vi "GXMLTest.vi"() -> ()   [LabVIEW 2015]
uses:
  <vilib>/NI/GXML/_subVIs/GXML SearchParser/Search Parser.vi
  <vilib>/NI/GXML/GXML.lvlib
panel:
  in  "Write?":bool
  in  "XML File Path":path=path "C:/SoftwareDevelopment/Workspace_2017/XpathTest/src/xpathTest/gxmlExport.xml"
  out "Concatenated GXML String":string
  in  "PID":T1
  in  "encoder":T2
  in  "limit":T3
  in  "template":T4
  in  "motor":T5
  in  "xmlEntries":enum32{"IntakeLift", "ChooChoo"}(tab)
  in  "IntakeLift":T4
  in  "ChooChoo":T4
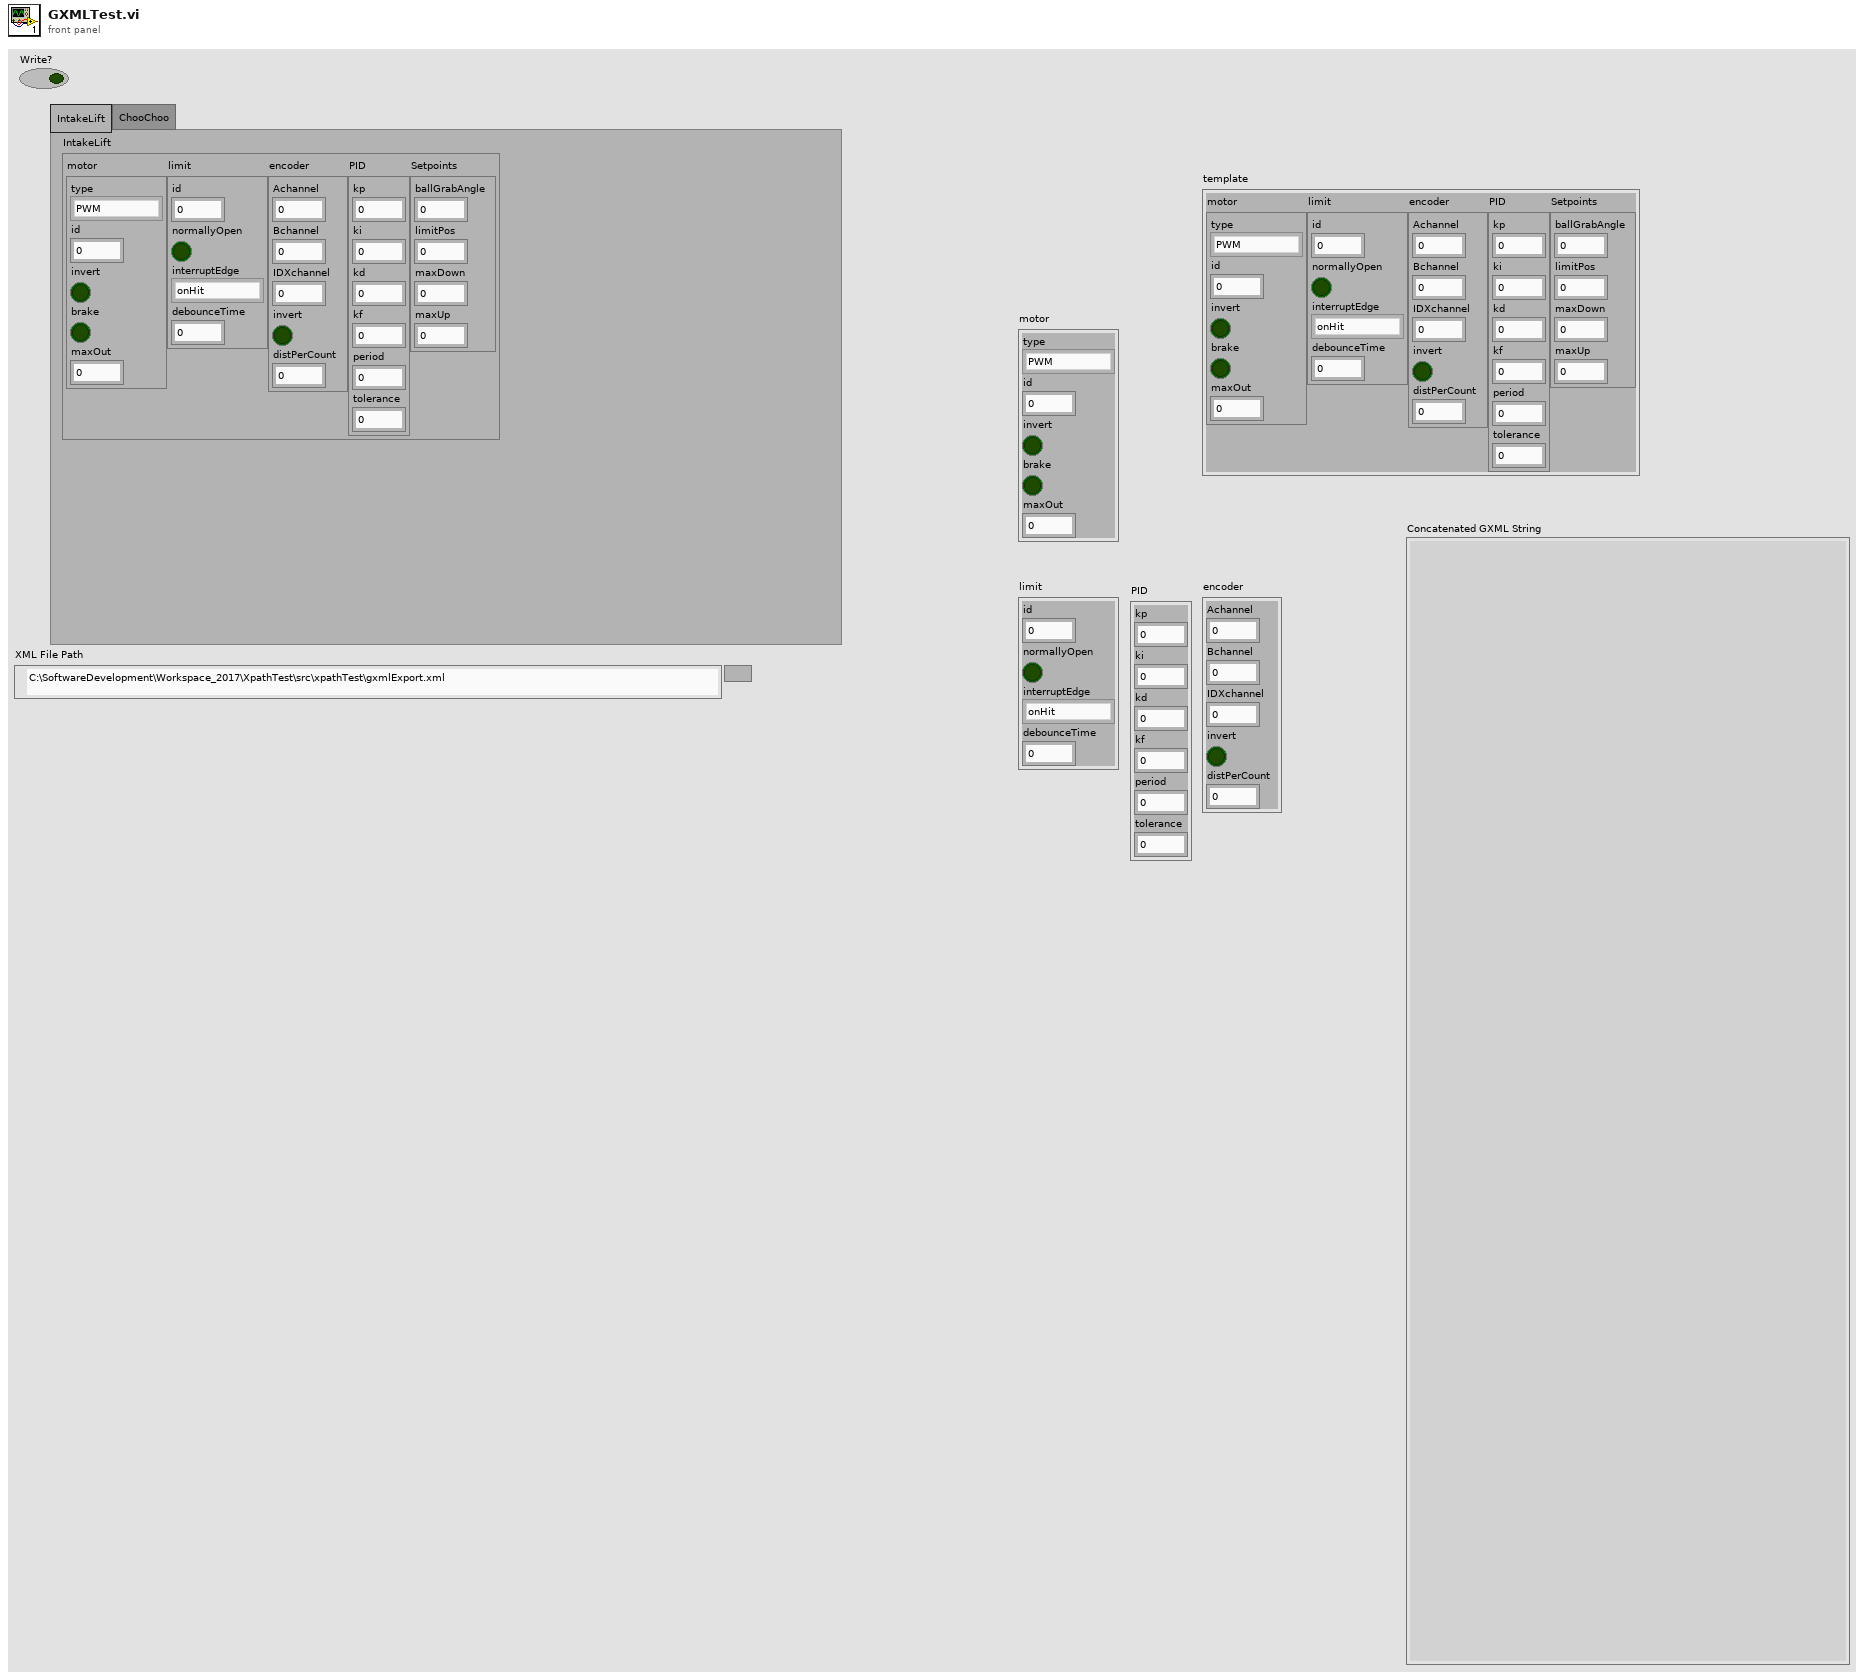
[diagram p1: front panel]
types:
  T1 = cluster{"kp":dbl, "ki":dbl, "kd":dbl, "kf":dbl, "period":dbl, "tolerance":dbl}
  T2 = cluster{"Achannel":i32, "Bchannel":i32, "IDXchannel":i32, "invert":bool, "distPerCount":dbl}
  T3 = cluster{"id":i32, "normallyOpen":bool, "interruptEdge":enum16{"onHit", "onRelease", "both"}, "debounceTime":dbl}
  T4 = cluster{"motor":cluster{"type":enum16{"PWM", "CANTalon"}, "id":i32, "invert":bool, "brake":bool, "maxOut":dbl}, "limit":cluster{"id":i32, "normallyOpen":bool, "interruptEdge":enum16{"onHit", "onRelease", "both"}, "debounceTime":dbl}, "encoder":cluster{"Achannel":i32, "Bchannel":i32, "IDXchannel":i32, "invert":bool, "distPerCount":dbl}, "PID":cluster{"kp":dbl, "ki":dbl, "kd":dbl, "kf":dbl, "period":dbl, "tolerance":dbl}, "Setpoints":cluster{"ballGrabAngle":dbl, "limitPos":dbl, "maxDown":dbl, "maxUp":dbl}}
  T5 = cluster{"type":enum16{"PWM", "CANTalon"}, "id":i32, "invert":bool, "brake":bool, "maxOut":dbl}
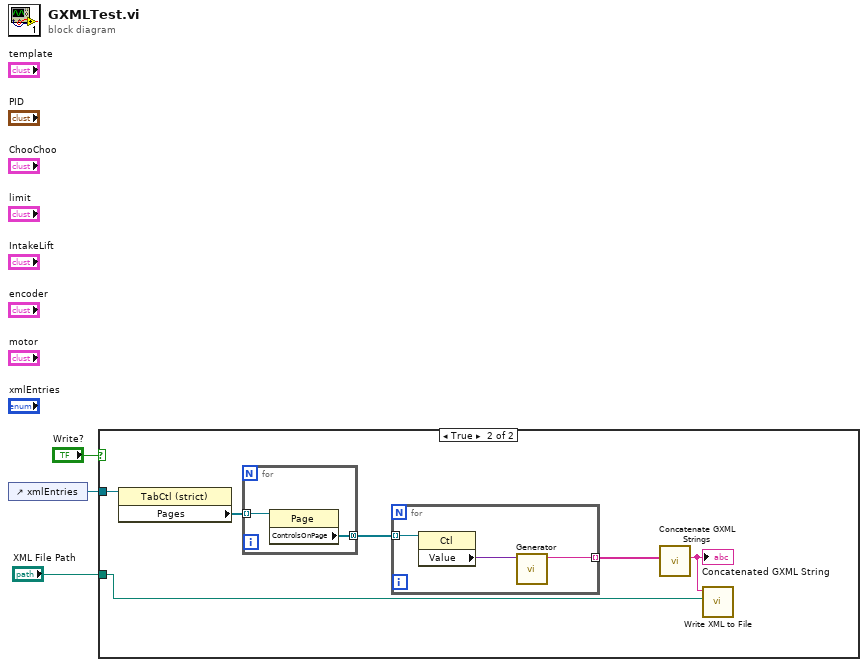
[diagram p0: block diagram]
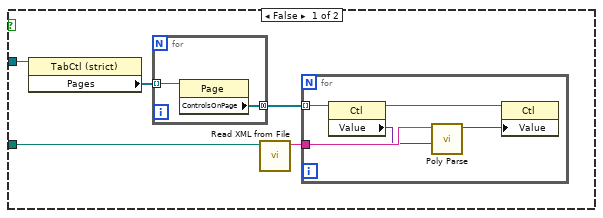
[diagram p2: hidden frame]
diagram:
  n1 = control-ref of="xmlEntries"() -> (w1:refnum<vi>)
  n2 = case shown="True" "Write?" {
    tunnel: "XML File Path" -> [w5 w17]
    tunnel: w1 -> [w6 w16]
    frame False {
      n3 = property class="TabCtl (strict)"(reference=w6) -> ("Pages"=w8:refnum<vi>[])  [unwired: 1 in, 2 out]
      n4 = for {
        tunnel: w8 -> [w15] mode=indexing
        tunnel: [w14] -> w7 mode=concatenating
        n5 = property class="Page"(reference=w15) -> ("ControlsOnPage"=w14:refnum<vi>[])  [unwired: 1 in, 2 out]
      }
      n6 = call <vilib>:"Read XML from File.vi"("XML File Path"=w5) -> ("XML String Out"=w4:string)  [unwired: 9 in, 1 out]
      n7 = for {
        tunnel: w7 -> [w13] mode=indexing
        tunnel: w4 -> [w12]
        n8 = property class="Ctl"(reference=w13) -> (reference out=w9:refnum<vi>, "Value"=w11:variant)  [unwired: 1 in, 1 out]
        n9 = call-poly <vilib>:"Poly Parse.vi"("TypeDesc"=w11, "XML String In"=w12) -> ("Parsed Data"=w10:variant)  [unwired: 8 in, 1 out]
        n10 = property class="Ctl"(reference=w9, "Value"=w10) -> ()  [unwired: 1 in, 2 out]
      }
    }
    frame True {
      n11 = property class="TabCtl (strict)"(reference=w16) -> ("Pages"=w21:refnum<vi>[])  [unwired: 1 in, 2 out]
      n12 = for {
        tunnel: w21 -> [w26] mode=indexing
        tunnel: [w25] -> w20 mode=concatenating
        n13 = property class="Page"(reference=w26) -> ("ControlsOnPage"=w25:refnum<vi>[])  [unwired: 1 in, 2 out]
      }
      n14 = for {
        tunnel: w20 -> [w24] mode=indexing
        tunnel: [w22] -> w19 mode=indexing
        n15 = property class="Ctl"(reference=w24) -> ("Value"=w23:variant)  [unwired: 1 in, 2 out]
        n16 = call <vilib>:"Generator.vi"("Variant"=w23) -> ("XML String Out"=w22:string)  [unwired: 9 in, 1 out]
      }
      n17 = call <vilib>:"Concatenate GXML Strings.vi"("GXML Strings"=w19) -> ("Concatenated GXML String"=w18:string)  [unwired: 9 in, 1 out]
      "Concatenated GXML String" <- w18
      n18 = call <vilib>:"Write XML to File.vi"("XML File Path"=w17, "XML Input"=w18) -> ()  [unwired: 9 in, 1 out]
    }
  }
